vi "tester.vi"() -> ()   [LabVIEW 2025]
uses:
  <vilib>/Utility/file.llb/Write Delimited Spreadsheet (string).vi
  <vilib>/Utility/file.llb/Write Delimited Spreadsheet (DBL).vi
panel:
  out "date/time string":string
  out "Array":string[](array[string])
  in  "All Counts":T1(graph)
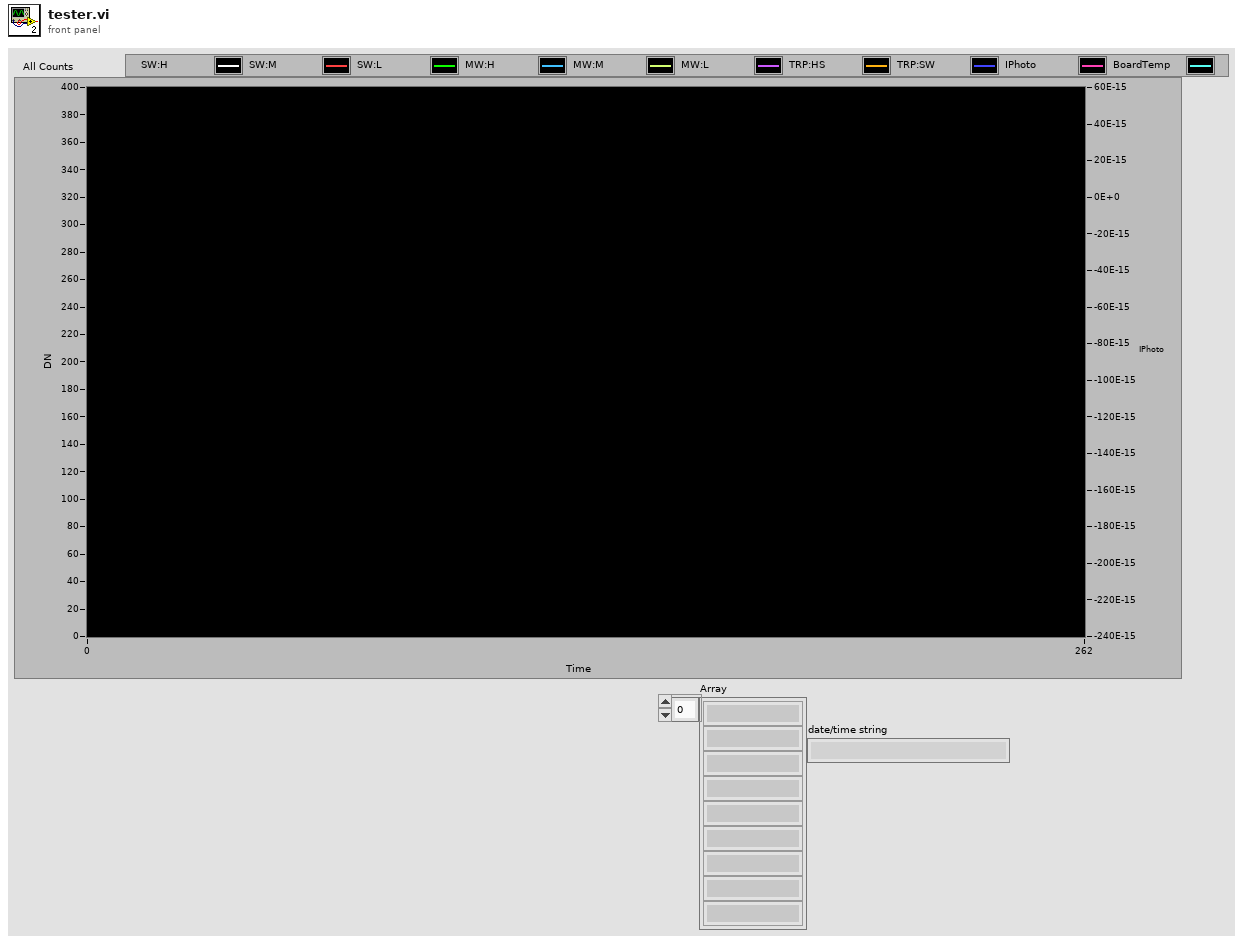
[diagram p1: front panel]
types:
  T1 = cluster{"[0]":dbl, "[1]":dbl, "[2]":dbl, "[3]":dbl, "[4]":dbl, "[5]":dbl, "[6]":dbl, "[7]":dbl, "[8]":dbl, "[9]":dbl}
  T2 = cluster{"[0]":dbl, "[1]":dbl, "[2]":dbl, "[3]":dbl, "[4]":dbl, "[5]":dbl, "[6]":dbl, "[7]":dbl, "[8]":dbl, "[9]":dbl}[]
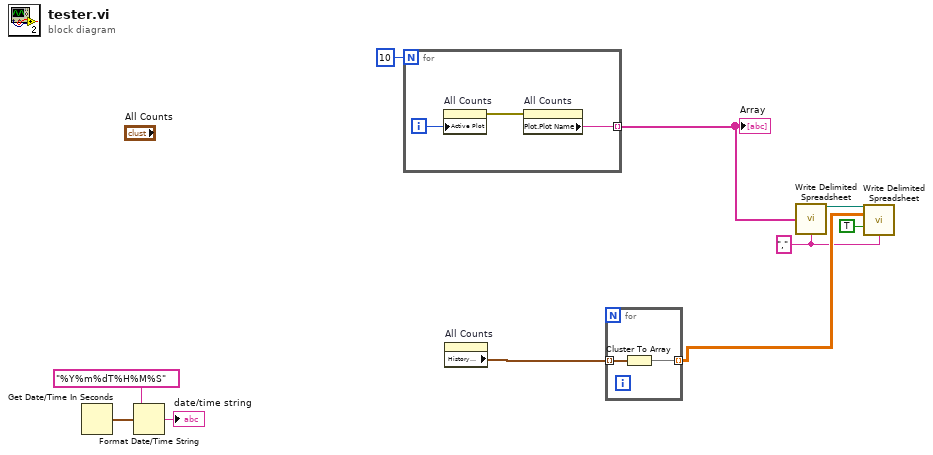
[diagram p0: block diagram]
diagram:
  w4 = "," ("delimiter (\\t)")
  n1 = Get Date/Time In Seconds() -> (seconds since 1Jan1904=w3:timestamp)
  n2 = Format Date/Time String(time format string (%c)="%Y%m%dT%H%M%S", seconds (now)=w3) -> (date/time string=→"date/time string":string)  [unwired: 1 in]
  n3 = for {
    N: 10 -> [_]
    tunnel: [w11] -> w8 mode=indexing
    i -> [w13]
    n4 = property on="All Counts" class="WFChart (strict)"("Active Plot"=w13) -> (error out=w12:errorcluster)  [unwired: 2 in, 1 out]
    n5 = property on="All Counts" class="WFChart (strict)"(error in=w12) -> ("Plot.Plot Name"=w11:string)  [unwired: 1 in, 2 out]
  }
  "Array" <- w8
  n6 = property on="All Counts" class="WFChart (strict)"() -> ("History Data"=w9:T2)  [unwired: 2 in, 2 out]
  n7 = for {
    tunnel: w9 -> [w15] mode=indexing
    tunnel: [w14] -> w6 mode=indexing
    n8 = Cluster To Array(cluster=w15) -> (array=w14:dbl[])
  }
  n9 = call-poly <vilib>:"Write Delimited Spreadsheet.vi"("1D data"=w8, "delimiter (\\t)"=w4) -> ("new file path (Not A Path if cancelled)"=w7:path)  [unwired: 12 in, 1 out]
  n10 = call-poly <vilib>:"Write Delimited Spreadsheet.vi"("file path (dialog if empty)"=w7, "2D data"=w6, "append to file? (new file:F)"=TRUE, "delimiter (\\t)"=w4) -> ()  [unwired: 10 in, 2 out]
